vi "日報表.vi"(9 "End Date":string="2014/10/03") -> (0 "error out 2":errorcluster)   [LabVIEW 2012]
uses:
  <vilib>/Utility/NIReport.llb/NI_report.lvclass
  Global1.vi
  <vilib>/Utility/NIReport.llb/Append Text Table to Report (wrap).vi
  <vilib>/Utility/NIReport.llb/Excel/NI_Excel.lvclass
  <vilib>/addons/_office/NI_ReportGenerationToolkit.lvlib
panel:
  in  "MonthToDate":string[][](array[string])
  out "Row Headers":string[](array[string])
  in  "Summary":string[][](array[string])
  in  "ShiftC":string[][](array[string])
  in  "ShiftB":string[][](array[string])
  in  "ShiftA":string[][](array[string])
  out "error out":errorcluster
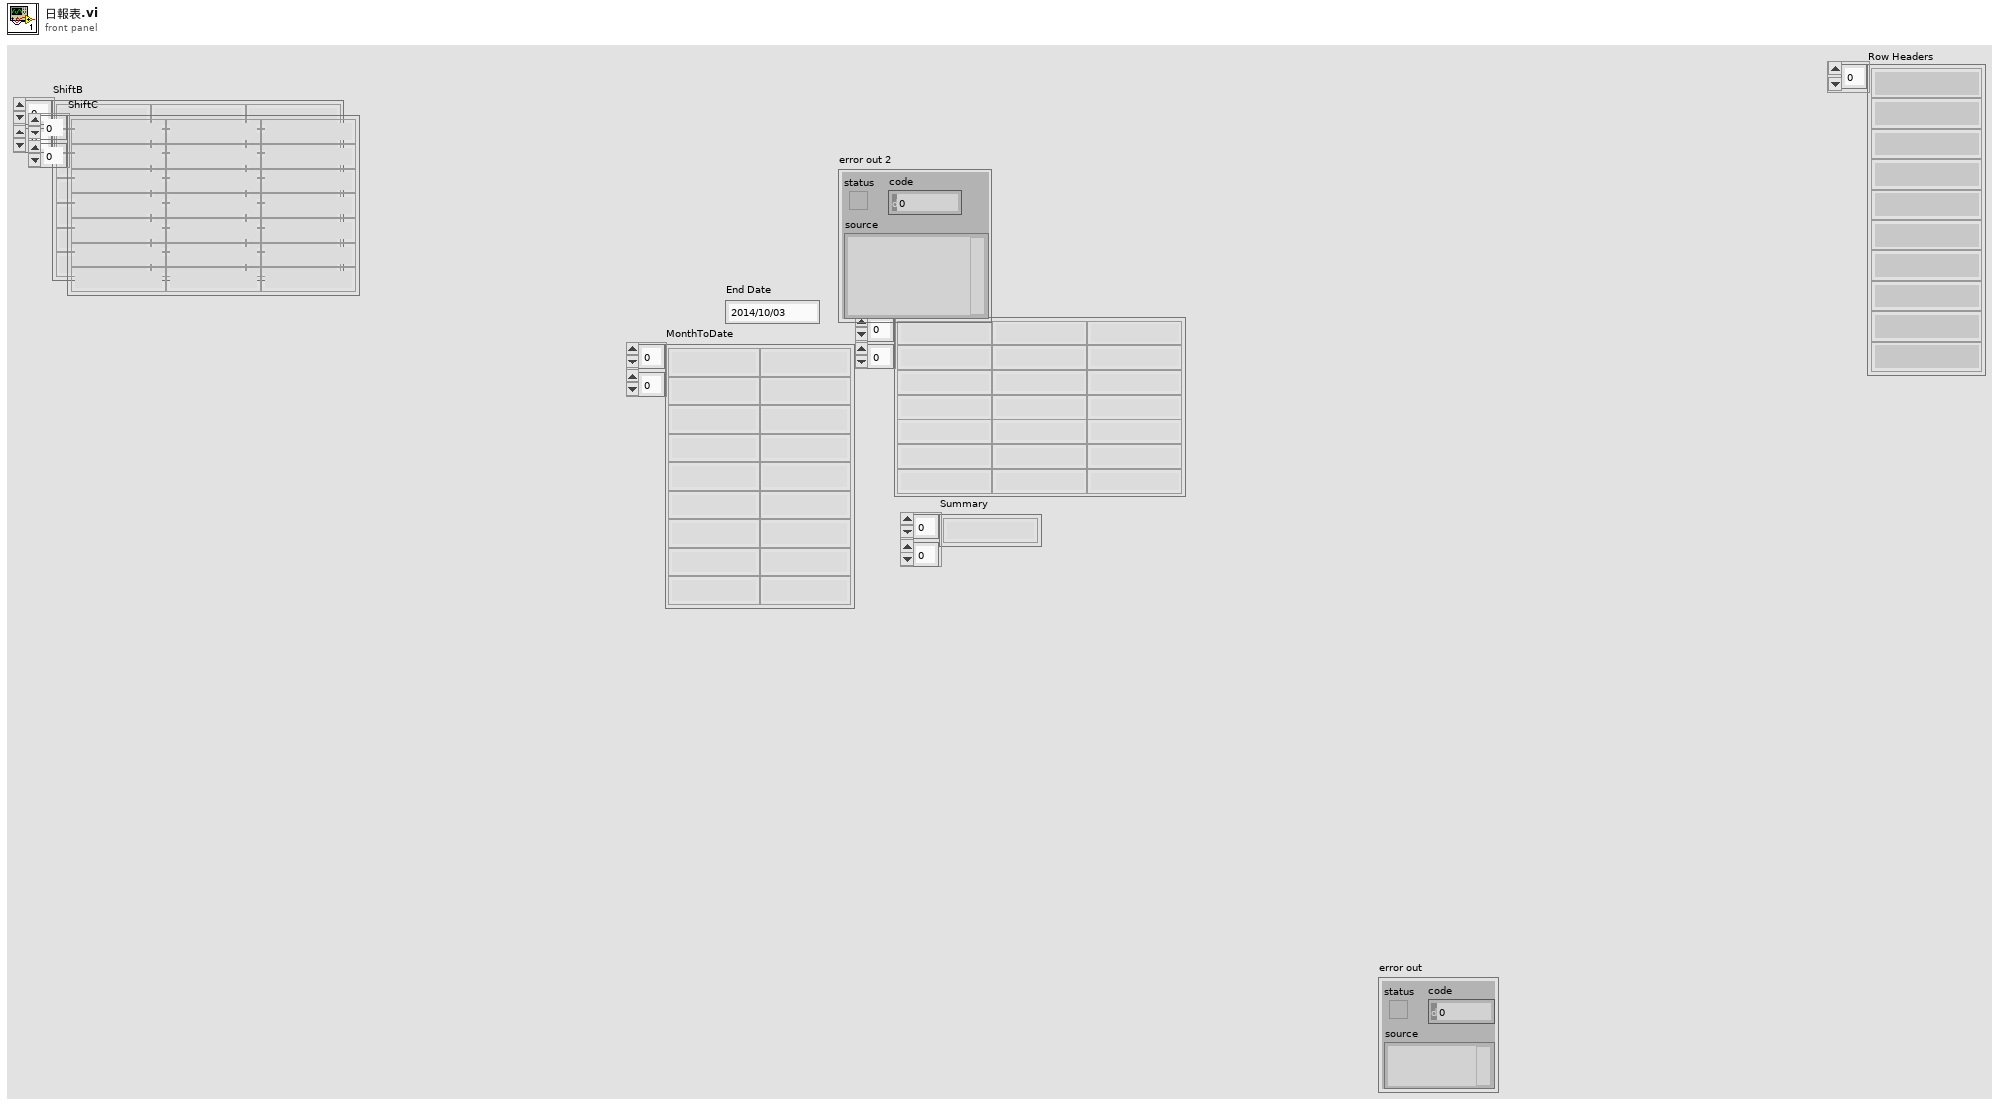
[diagram p1: front panel]
types:
  T1 = enum16{"Standard Report", "HTML", "Word", "Excel"}
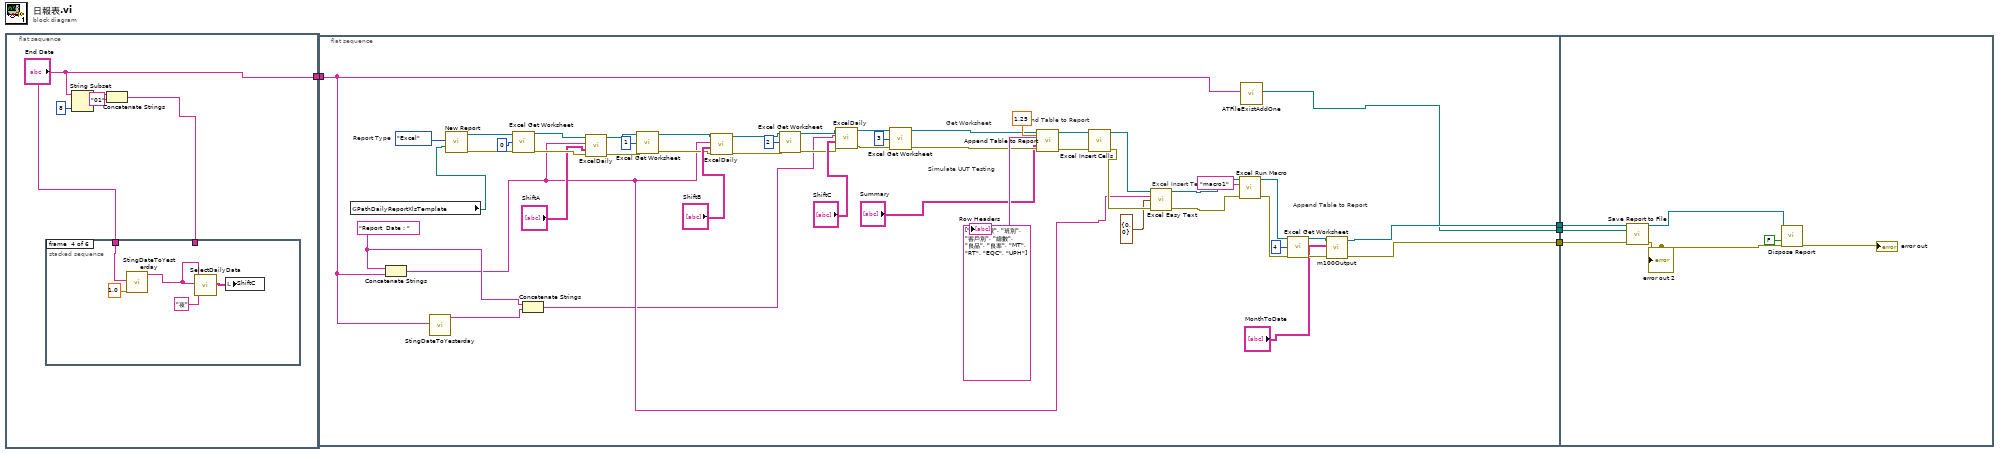
[diagram p0: block diagram]
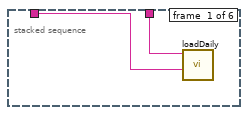
[diagram p2: hidden frame]
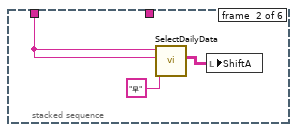
[diagram p3: hidden frame]
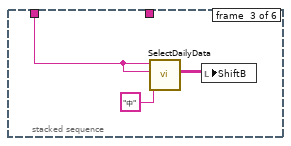
[diagram p4: hidden frame]
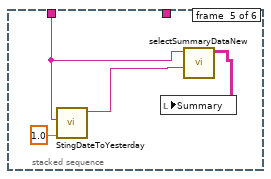
[diagram p5: hidden frame]
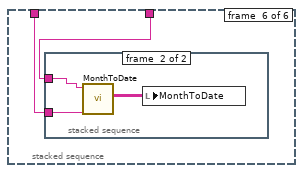
[diagram p6: hidden frame]
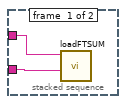
[diagram p7: hidden frame]
diagram:
  n1 = flat-sequence {
    tunnel: ["End Date"] -> w4
    frame #0 {
      n2 = String Subset(string="End Date", length (rest)=8 ("length (rest)")) -> (substring=w8:string)  [unwired: 1 in]
      n3 = Concatenate Strings(w8, "01" ("string")) -> (w6:string)
      n4 = stacked-sequence {
        tunnel: w6 -> [w10 _ _ _ _ w27]
        tunnel: "End Date" -> [w11 w12 w15 w20 w25 w28]
        frame #0 {
          n5 = call "loadDaily.vi"("end date"=w11, "begin date"=w10) -> ()  [unwired: 9 in, 1 out]
        }
        frame #1 {
          n6 = call "SelectDailyData.vi"("Shift"="早", "Begin_date"=w12, "End_date"=w12) -> ("output array"=w13:string[][])  [unwired: 8 in]
          n7 = local write "ShiftA"(w13) -> ()
        }
        frame #2 {
          n8 = call "SelectDailyData.vi"("Shift"="中", "Begin_date"=w15, "End_date"=w15) -> ("output array"=w16:string[][])  [unwired: 8 in]
          n9 = local write "ShiftB"(w16) -> ()
        }
        frame #3 {
          n10 = call "StingDateToYesterday.vi"("Days"=1.0, "Date"=w20) -> ("Date+1"=w18:string)  [unwired: 8 in, 1 out]
          n11 = call "SelectDailyData.vi"("Shift"="夜", "Begin_date"=w18, "End_date"=w18) -> ("output array"=w21:string[][])  [unwired: 8 in]
          n12 = local write "ShiftC"(w21) -> ()
        }
        frame #4 {
          n13 = call "StingDateToYesterday.vi"("Days"=1.0, "Date"=w25) -> ("Date+1"=w24:string)  [unwired: 8 in, 1 out]
          n14 = call "selectSummaryDataNew.vi"("End Date"=w24, "From Date"=w25) -> ("Summary"=w23:string[][])  [unwired: 9 in]
          n15 = local write "Summary"(w23) -> ()
        }
        frame #5 {
          n16 = stacked-sequence {
            tunnel: w28 -> [w30 w31]
            tunnel: w27 -> [w29 w32]
            frame #0 {
              n17 = call "loadFTSUM.vi"("End Date"=w30, "From Date"=w29) -> ()  [unwired: 9 in, 1 out]
            }
            frame #1 {
              n18 = call "MonthToDate.vi"("End Date"=w31, "From Date"=w32) -> ("output array"=w33:string[][])  [unwired: 8 in, 1 out]
              n19 = local write "MonthToDate"(w33) -> ()
            }
          }
        }
      }
    }
  }
  n20 = flat-sequence {
    tunnel: w4 -> [w38]
    tunnel: [w41] -> w3
    tunnel: [w40] -> w2
    tunnel: [w39] -> w1
    tunnel: w3 -> [w90]
    tunnel: w2 -> [w89]
    tunnel: w1 -> [w88]
    frame #0 {
      w36 = "Report  Date : " ("string")
      w60 = string[] ["機台編號", "班別", "客戶別", "總數", "良品", "良率", "MT", "RT", "EQC", "UPH"] ("row headers")
      w83 = T1."Excel"  # Report Type
      # "Append Table to Report"
      # "Excel Insert Text"
      # "Simulate UUT Testing"
      # "Append Table to Report"
      # "Get Worksheet"
      n21 = global read "Global1.vi" "PathDailyReportXlsTemplate"() -> (w42:path)
      n22 = Concatenate Strings(w36, w38) -> (w35:string)
      n23 = call "StingDateToYesterday.vi"("Date"=w38) -> ("Date+1"=w37:string)  [unwired: 9 in, 1 out]
      n24 = call <vilib>:"New Report.vi"("report type"=w83, "template (empty)"=w42) -> ("report out"=w82:refnum<class "NI_report.lvclass">, "error out"=w81:errorcluster)  [unwired: 12 in]
      n25 = call <vilib>:"Excel Get Worksheet.vi"("report in"=w82, "worksheet index (0)"=0, "error in (no error)"=w81) -> ("report out"=w79:refnum<class "NI_report.lvclass">, "error out"=w78:errorcluster)  [unwired: 11 in]
      n26 = Concatenate Strings(w36, w37) -> (w34:string)
      n27 = call "ExcelDaily.vi"("error in (no error)"=w78, "Input"="ShiftA", "Header"=w35, "report in"=w79) -> ("error out"=w72:errorcluster, "report out"=w74:refnum<class "NI_report.lvclass">)  [unwired: 6 in]
      n28 = call <vilib>:"Excel Get Worksheet.vi"("report in"=w74, "worksheet index (0)"=1, "error in (no error)"=w72) -> ("report out"=w73:refnum<class "NI_report.lvclass">, "error out"=w71:errorcluster)  [unwired: 11 in]
      n29 = call "ExcelDaily.vi"("error in (no error)"=w71, "Input"="ShiftB", "Header"=w35, "report in"=w73) -> ("error out"=w68:errorcluster, "report out"=w69:refnum<class "NI_report.lvclass">)  [unwired: 6 in]
      n30 = call <vilib>:"Excel Get Worksheet.vi"("report in"=w69, "worksheet index (0)"=2, "error in (no error)"=w68) -> ("report out"=w67:refnum<class "NI_report.lvclass">, "error out"=w66:errorcluster)  [unwired: 11 in]
      n31 = call "ExcelDaily.vi"("error in (no error)"=w66, "Input"="ShiftC", "Header"=w34, "report in"=w67) -> ("error out"=w63:errorcluster, "report out"=w64:refnum<class "NI_report.lvclass">)  [unwired: 6 in]
      n32 = call <vilib>:"Excel Get Worksheet.vi"("report in"=w64, "worksheet index (0)"=3, "error in (no error)"=w63) -> ("report out"=w51:refnum<class "NI_report.lvclass">, "error out"=w50:errorcluster)  [unwired: 11 in]
      n33 = call-poly <vilib>:"Append Table to Report.vi"("report in"=w51, "column width (1)"=1.25, "column headers"=w60, "text data"="Summary", "error in (no error)"=w50) -> ("report out"=w59:refnum<class "NI_report.lvclass">, "error out"=w58:errorcluster)  [unwired: 7 in, 2 out]
      n34 = call <vilib>:"Excel Insert Cells.vi"("report in"=w59, "error in (no error)"=w58) -> ("report out"=w57:refnum<class "NI_report.lvclass">, "error out"=w56:errorcluster)  [unwired: 12 in]
      n35 = call <vilib>:"Excel Easy Text.vi"("report in"=w57, "text"=w35, "start (-1, -1)"=cluster{"row":i32, "column":i32} {"row"=0, "column"=0} ("end (-1, -1)"), "error in (no error)"=w56) -> ("report out"=w54:refnum<class "NI_report.lvclass">, "error out"=w53:errorcluster)  [unwired: 7 in, 3 out]
      n36 = call <vilib>:"Excel Run Macro.vi"("report in"=w54, "macro name"="macro1", "error in (no error)"=w53) -> ("report out"=w48:refnum<class "NI_report.lvclass">, "error out"=w47:errorcluster)  [unwired: 10 in, 1 out]
      n37 = call "ATFileExistAddOne.vi"("input string"=w38) -> ("appended path"=w39:path)  [unwired: 10 in]
      n38 = call <vilib>:"Excel Get Worksheet.vi"("report in"=w48, "worksheet index (0)"=4, "error in (no error)"=w47) -> ("report out"=w45:refnum<class "NI_report.lvclass">, "error out"=w44:errorcluster)  [unwired: 11 in]
      n39 = call "m100Output.vi"("error in (no error)"=w44, "Input"="MonthToDate", "report in"=w45) -> ("error out"=w40:errorcluster, "report out"=w41:refnum<class "NI_report.lvclass">)  [unwired: 7 in]
      "Row Headers" <- w60
    }
    frame #1 {
      n40 = call-dynamic "Save Report to File.vi"("report in"=w90, "report file path"=w88, "error in (no error)"=w89) -> ("report out"=w87:refnum<class "NI_report.lvclass">, "error out"=w86:errorcluster)  [unwired: 11 in]
      "error out 2" <- w86
      n41 = call-dynamic "Dispose Report.vi"("report in"=w87, "save changes? (F)"=FALSE, "error in (no error)"=w86) -> ("error out"=→"error out":errorcluster)  [unwired: 12 in]
    }
  }
